vi "EnableDisable RTM.vi"(8 "error in (no error)":errorcluster, 11 "Node Ptr":u64 format="%.0x") -> (0 "error out":errorcluster)   [LabVIEW 2020, in "Ballard MIL-STD-1553 System Explorer.lvlib" / "Implementation.lvlib"]
uses:
  Implementation.lvlib
  Scripting/Ballard MIL-STD-1553 Scripting.lvlib
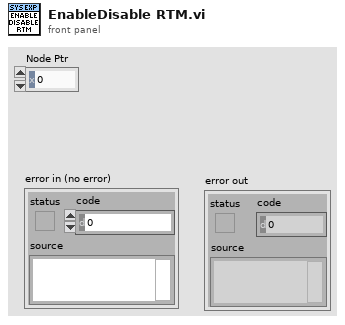
[diagram p1: front panel]
types:
  T1 = typedef "Custom Device API.lvlib/Custom Device Item Ref.ctl" = u64
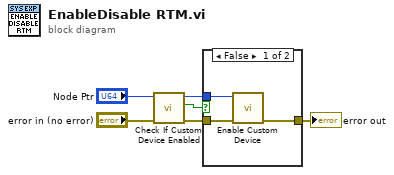
[diagram p0: block diagram]
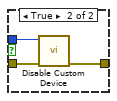
[diagram p2: hidden frame]
diagram:
  n1 = call "Check If Custom Device Enabled.vi"("error in"="error in (no error)", "Ballard MIL-STD 1553 custom device in"="Node Ptr") -> ("error out"=w3:errorcluster, "Is Custom Device Enabled?"=w5:bool, "Ballard MIL-STD 1553 custom device out"=w4:T1)  [unwired: 7 in]
  n2 = case shown="False" w5 {
    tunnel: w4 -> [w9 w12]
    tunnel: w3 -> [w8 w11]
    tunnel: [w7 w10] -> w2
    frame False {
      n3 = call "Enable Custom Device.vi"("error in"=w8, "Ballard MIL-STD 1553 custom device in"=w9) -> ("error out"=w7:errorcluster)  [unwired: 8 in, 1 out]
    }
    frame True {
      n4 = call "Disable Custom Device.vi"("error in"=w11, "Ballard MIL-STD 1553 custom device in"=w12) -> ("error out"=w10:errorcluster)  [unwired: 8 in, 1 out]
    }
  }
  "error out" <- w2
